vi "SP SP - set value STR.vi"(8 "error in (no error)":errorcluster, 11 "JSON string":string) -> (0 "error out":errorcluster, 3 "value":string)   [LabVIEW 2020, in "ui-testing.lvlib"]
doc: "copyright: Thomas Zilliox©"
uses:
  ui-testing.lvlib
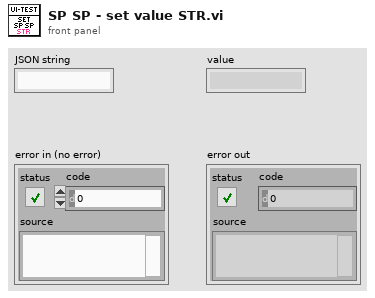
[diagram p1: front panel]
types:
  T1 = cluster{"control":string, "subpanel":string, "subsubpanel":string, "value":string}
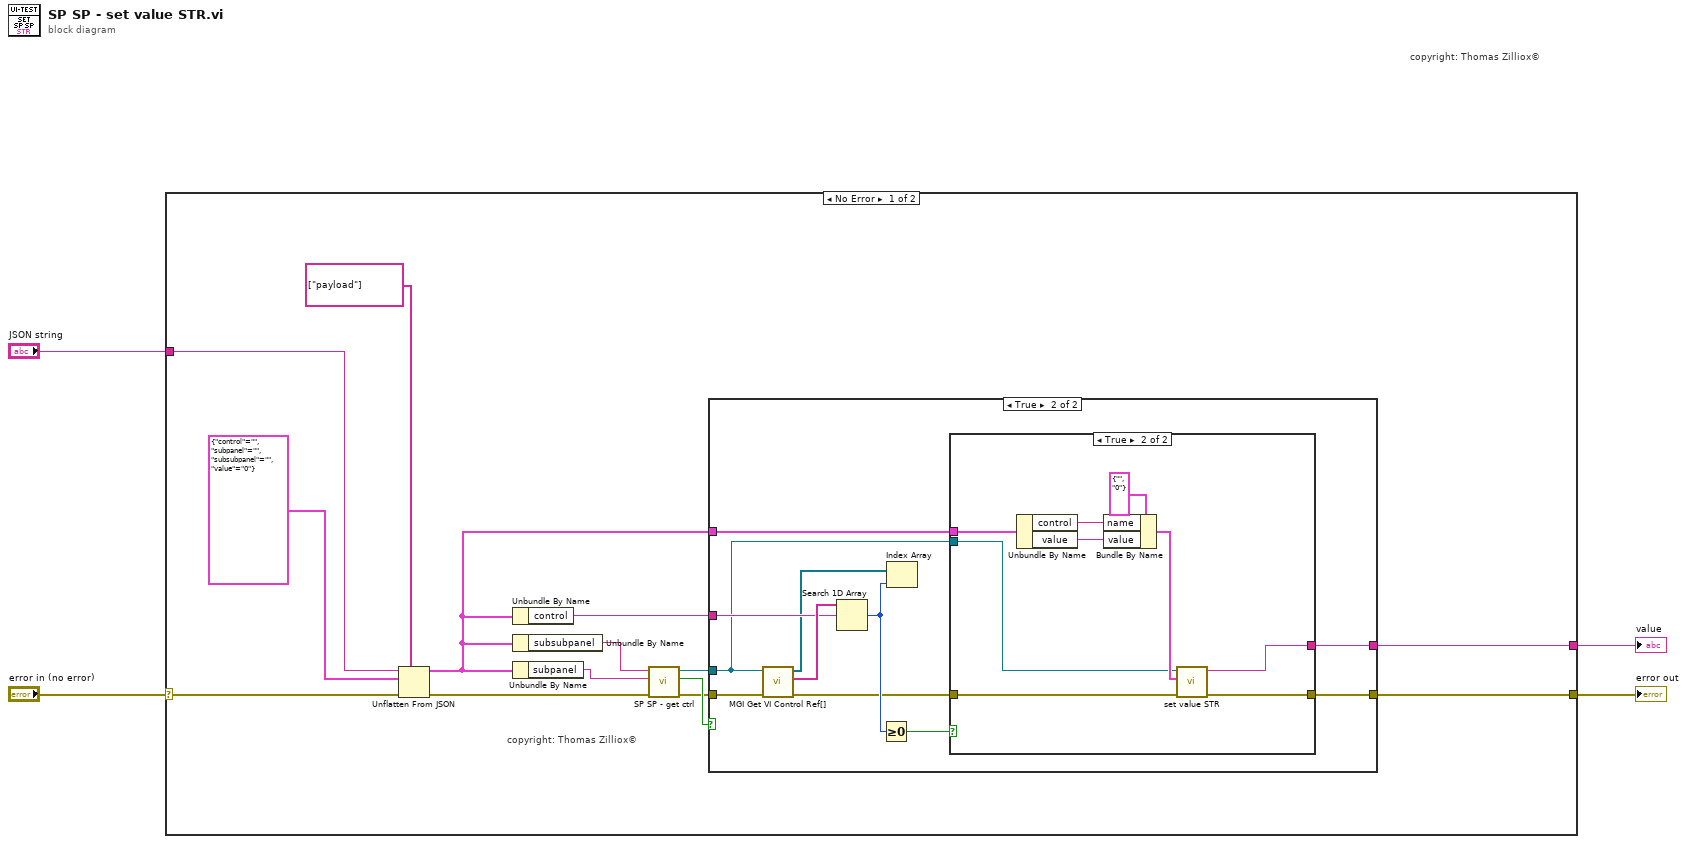
[diagram p0: block diagram]
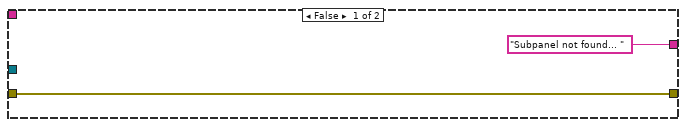
[diagram p2: hidden frame]
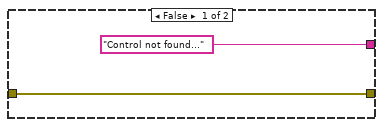
[diagram p3: hidden frame]
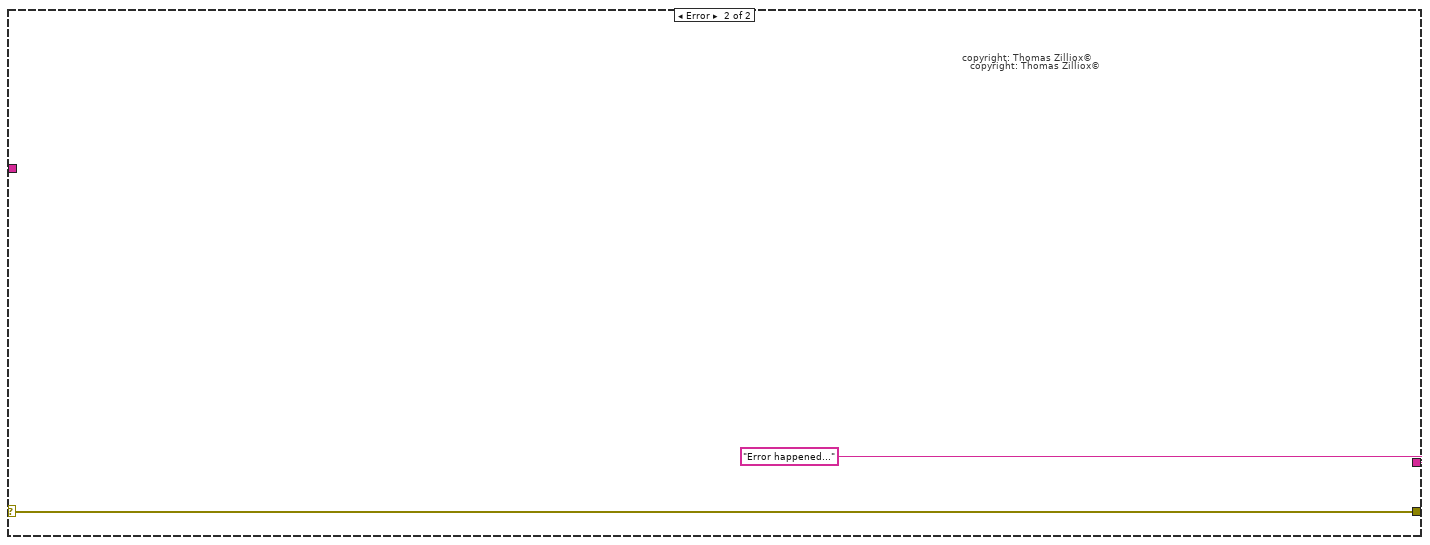
[diagram p4: hidden frame]
diagram:
  # "copyright: Thomas Zilliox©"
  n1 = case shown="No Error" "error in (no error)" {
    selector: "error in (no error)" -> [w14 w44]
    tunnel: "JSON string" -> [w16 _]
    tunnel: [w15 w44] -> w3
    tunnel: [w13 "Error happened..."] -> w1
    frame No Error {
      # "copyright: Thomas Zilliox©"
      n2 = Unflatten From JSON(path=string[] ["payload"], JSON string=w16, type and defaults=T1 {"control"="", "subpanel"="", "subsubpanel"="", "value"="0"}, error in (no error)=w14) -> (value=w6:T1, error out=w17:errorcluster)  [unwired: 3 in]
      n3 = Unbundle By Name(w6) -> ("control"=w9:string)
      n4 = Unbundle By Name(w6) -> ("subsubpanel"=w5:string)
      n5 = Unbundle By Name(w6) -> ("subpanel"=w12:string)
      n6 = call "SP SP - get ctrl.vi"("error in (no error)"=w17, "subpanel"=w12, "subsubpanel"=w5) -> ("error out"=w7:errorcluster, "Boolean"=w8:bool, "VI out"=w10:refnum<vi>)  [unwired: 6 in]
      n7 = case shown="True" w8 {
        tunnel: [w20 w31] -> w15
        tunnel: w10 -> [_ w21]
        tunnel: w7 -> [w20 w29]
        tunnel: w9 -> [_ w27]
        tunnel: ["Subpanel not found... " ("result string") w30] -> w13
        tunnel: w6 -> [_ w22]
        frame False {
        }
        frame True {
          n8 = call <userlib>:"MGI Get VI Control Ref[].vi"("error in"=w29, "VI (Caller)"=w21) -> ("error out"=w24:errorcluster, "Control Label Chain[i]"=w28:string[], "Control[i]"=w26:refnum<vi>[])  [unwired: 6 in, 1 out]
          n9 = Search 1D Array(1D array=w28, element=w27) -> (index of element=w25:i32)  [unwired: 1 in]
          n10 = Greater Or Equal To 0?(x=w25) -> (x >= 0?=w23:bool)
          n11 = Index Array(array=w26, index=w25) -> ()  [unwired: 1 out]
          n12 = case shown="True" w23 {
            tunnel: w24 -> [w33 w36]
            tunnel: [w33 w34] -> w31
            tunnel: ["Control not found..." ("result string") w35] -> w30
            tunnel: w22 -> [_ w38]
            tunnel: w21 -> [_ w37]
            frame False {
            }
            frame True {
              n13 = Unbundle By Name(w38) -> ("control"=w39:string, "value"=w40:string)
              n14 = Bundle By Name(cluster=cluster{"name":string, "value":string} {"name"="", "value"="0"} ("Payload"), "name"=w39, "value"=w40) -> (w41:cluster{"name":string, "value":string})
              n15 = call "set value STR.vi"("error in (no error)"=w36, "Payload"=w41, "VI Ref"=w37) -> ("error out"=w34:errorcluster, "return value"=w35:string)  [unwired: 7 in]
            }
          }
        }
      }
    }
    frame Error {
      # "copyright: Thomas Zilliox©"
      # "copyright: Thomas Zilliox©"
    }
  }
  "error out" <- w3
  "value" <- w1
